vi "Operator Input click on 1 of 3 choices.vi"(7 "button3 text":string, 8 "error in (no error)":errorcluster, 9 "button2 text":string, 10 "button1 text":string, 11 "Operator text":string) -> (0 "error out":errorcluster, 1 "button3 clicked?":bool, 2 "button2 clicked?":bool, 3 "button1 clicked?":bool)   [LabVIEW 2013]
panel:
  in  "button3 clicked":bool caption="button3 clicked?"
  in  "button2 clicked":bool caption="button2 clicked?"
  in  "button1 clicked":bool caption="button1 clicked?"
  out "Message":string
  # "Operator Message"
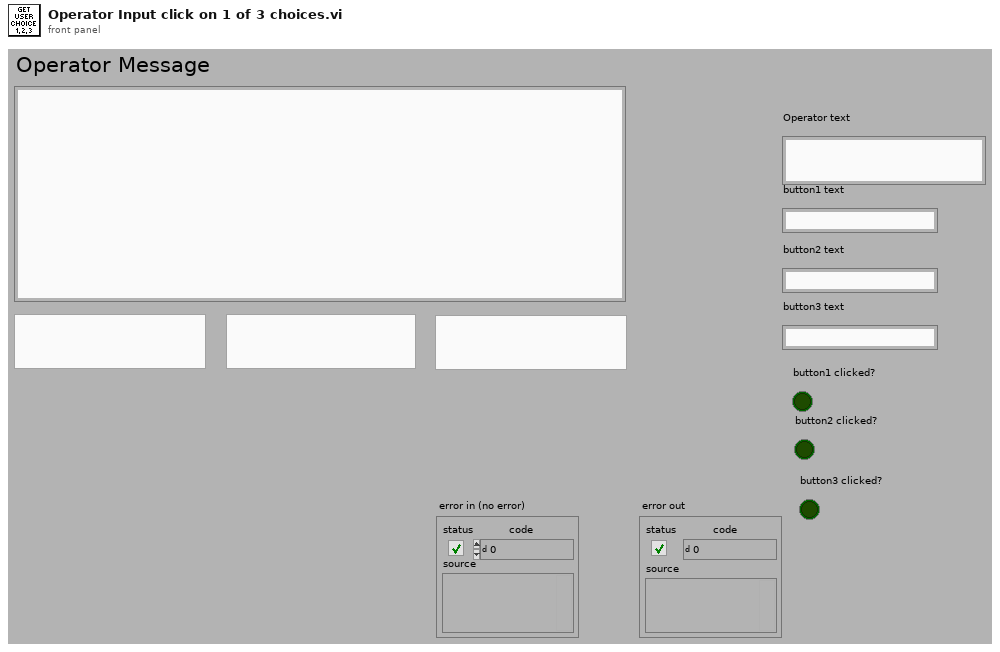
[diagram p1: front panel]
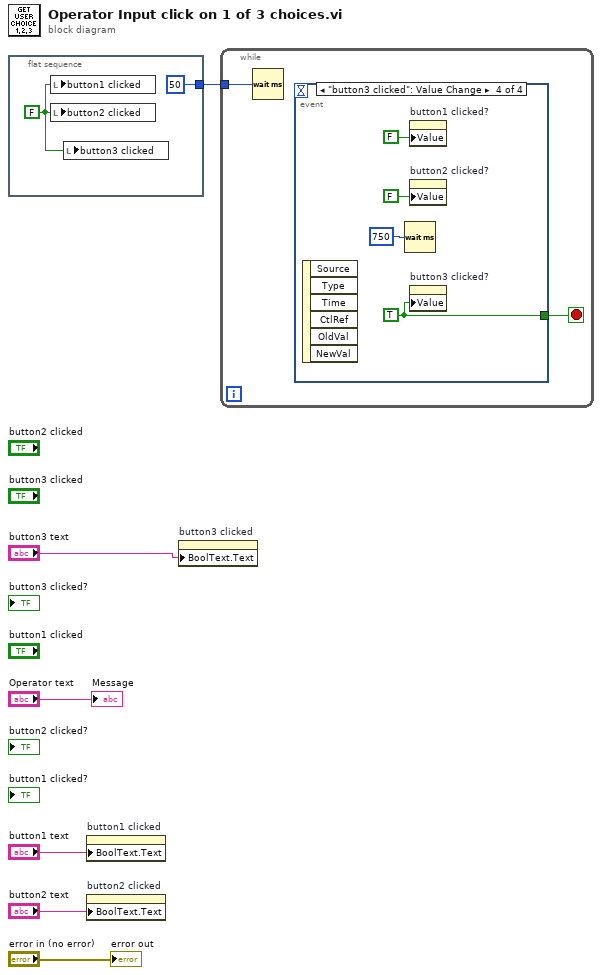
[diagram p0: block diagram]
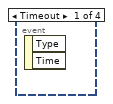
[diagram p2: hidden frame]
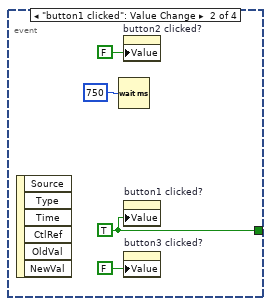
[diagram p3: hidden frame]
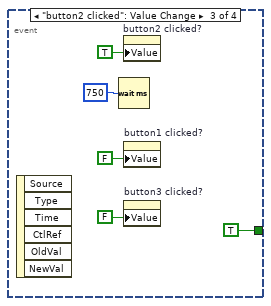
[diagram p4: hidden frame]
diagram:
  n1 = flat-sequence {
    tunnel: [u32 50 ("milliseconds to wait")] -> w6
    frame #0 {
      w7 = FALSE ("button1")
      n2 = local write "button1 clicked"(w7) -> ()
      n3 = local write "button2 clicked"(w7) -> ()
      n4 = local write "button3 clicked"(w7) -> ()
    }
  }
  n5 = property on="button1 clicked" class="Bool (strict)"("BoolText.Text"="button1 text") -> ()  [unwired: 2 in, 2 out]
  n6 = property on="button2 clicked" class="Bool (strict)"("BoolText.Text"="button2 text") -> ()  [unwired: 2 in, 2 out]
  n7 = property on="button3 clicked" class="Bool (strict)"("BoolText.Text"="button3 text") -> ()  [unwired: 2 in, 2 out]
  n8 = while {
    tunnel: w6 -> [w10]
    stop <- w9 stop-if-true
    n9 = Wait (ms)(milliseconds to wait=w10) -> ()  [unwired: 1 out]
    n10 = event shown="[3] \"button3 clicked\": Value Change" {
      selector: _ -> [_ _ _ _]
      dyn-events: _ -> [_ _ _ _]
      timeout: _ -> [_ _ _ _]
      tunnel: [_ w14 TRUE w20] -> w9
      event Timeout {
        n11 = event-data() -> ()  [unwired: 1 in, 2 out]
      }
      event "button1 clicked": Value Change {
        w14 = TRUE
        n12 = event-data() -> ()  [unwired: 1 in, 6 out]
        n13 = Wait (ms)(milliseconds to wait=u32 750) -> ()  [unwired: 1 out]
        n14 = property on="button2 clicked?" class="Bool (strict)"("Value"=FALSE ("button2 clicked?")) -> ()  [unwired: 2 in, 2 out]
        n15 = property on="button1 clicked?" class="Bool (strict)"("Value"=w14) -> ()  [unwired: 2 in, 2 out]
        n16 = property on="button3 clicked?" class="Bool (strict)"("Value"=FALSE ("button3 clicked?")) -> ()  [unwired: 2 in, 2 out]
      }
      event "button2 clicked": Value Change {
        n17 = event-data() -> ()  [unwired: 1 in, 6 out]
        n18 = Wait (ms)(milliseconds to wait=u32 750) -> ()  [unwired: 1 out]
        n19 = property on="button2 clicked?" class="Bool (strict)"("Value"=TRUE ("button2 clicked?")) -> ()  [unwired: 2 in, 2 out]
        n20 = property on="button1 clicked?" class="Bool (strict)"("Value"=FALSE ("button1 clicked?")) -> ()  [unwired: 2 in, 2 out]
        n21 = property on="button3 clicked?" class="Bool (strict)"("Value"=FALSE ("button3 clicked?")) -> ()  [unwired: 2 in, 2 out]
      }
      event "button3 clicked": Value Change {
        w20 = TRUE ("button3 clicked?")
        n22 = event-data() -> ()  [unwired: 1 in, 6 out]
        n23 = Wait (ms)(milliseconds to wait=u32 750) -> ()  [unwired: 1 out]
        n24 = property on="button1 clicked?" class="Bool (strict)"("Value"=FALSE) -> ()  [unwired: 2 in, 2 out]
        n25 = property on="button2 clicked?" class="Bool (strict)"("Value"=FALSE ("button2 clicked?")) -> ()  [unwired: 2 in, 2 out]
        n26 = property on="button3 clicked?" class="Bool (strict)"("Value"=w20) -> ()  [unwired: 2 in, 2 out]
      }
    }
  }
  "Message" <- "Operator text"
  "error out" <- "error in (no error)"
